vi "transmit-8.6.vi"(0 "can卡类型":u8, 1 "设备索引号":u8, 2 "CAN端口":u8, 4 "单帧发送?":bool=TRUE, 5 "错误输入（无错误）":errorcluster, 6 "ID":u32 format="%x", 7 "SendType":u8, 8 "Data":u8[](array[numeric]), 9 "Eflag":u8=1 format="%x") -> (14 "返回值ID":u32 format="%x", 15 "发送返回值":u32, 16 "发送成功":bool, 19 "错误输出":errorcluster)   [LabVIEW 2013]
uses:
  AutoBurn/Settings/ControlCAN.dll
panel:
  in  "3":u8 format="%x"
  in  "2":u8 format="%x"
  in  "1":u8 format="%x"
  in  "长度":u8=8 format="%x"
  in  "RemoteFlag":u8 format="%x"
  in  "flag":u8 format="%x"
  in  "TimeStamp":u32 format="%x"
  out "VCI_CAN_OBJ_T":T1={"ID"=0, "TimeStamp"=0, "TimeFlag"=0, "SendType"=1, "RemoteFlag"=0, "ExternFlag"=0, "DataLen"=8, 0, 0, 0, 0, 0, 0, 0, 0, 0, 0, 0}
  in  "VCI_CAN_OBJ_T_N":T2(array[cluster])=[{"ID"=0, "TimeStamp"=0, "TimeFlag"=0, "SendType"=1, "RemoteFlag"=0, "ExternFlag"=0, "DataLen"=8, 0, 0, 0, 0, 0, 0, 0, 0, 0, 0, 0}, {"ID"=0, "TimeStamp"=0, "TimeFlag"=0, "SendType"=1, "RemoteFlag"=0, "ExternFlag"=0, "DataLen"=8, 0, 0, 0, 0, 0, 0, 0, 0, 0, 0, 0}, {"ID"=0, "TimeStamp"=0, "TimeFlag"=0, "SendType"=1, "RemoteFlag"=0, "ExternFlag"=0, "DataLen"=8, 0, 0, 0, 0, 0, 0, 0, 0, 0, 0, 0}, {"ID"=0, "TimeStamp"=0, "TimeFlag"=0, "SendType"=1, "RemoteFlag"=0, "ExternFlag"=0, "DataLen"=8, 0, 0, 0, 0, 0, 0, 0, 0, 0, 0, 0}, {"ID"=0, "TimeStamp"=0, "TimeFlag"=0, "SendType"=1, "RemoteFlag"=0, "ExternFlag"=0, "DataLen"=8, 0, 0, 0, 0, 0, 0, 0, 0, 0, 0, 0}, {"ID"=0, "TimeStamp"=0, "TimeFlag"=0, "SendType"=1, "RemoteFlag"=0, "ExternFlag"=0, "DataLen"=8, 0, 0, 0, 0, 0, 0, 0, 0, 0, 0, 0}, {"ID"=0, "TimeStamp"=0, "TimeFlag"=0, "SendType"=1, "RemoteFlag"=0, "ExternFlag"=0, "DataLen"=8, 0, 0, 0, 0, 0, 0, 0, 0, 0, 0, 0}, {"ID"=0, "TimeStamp"=0, "TimeFlag"=0, "SendType"=1, "RemoteFlag"=0, "ExternFlag"=0, "DataLen"=8, 0, 0, 0, 0, 0, 0, 0, 0, 0, 0, 0}, {"ID"=0, "TimeStamp"=0, "TimeFlag"=0, "SendType"=1, "RemoteFlag"=0, "ExternFlag"=0, "DataLen"=8, 0, 0, 0, 0, 0, 0, 0, 0, 0, 0, 0}, {"ID"=0, "TimeStamp"=0, "TimeFlag"=0, "SendType"=1, "RemoteFlag"=0, "ExternFlag"=0, "DataLen"=8, 0, 0, 0, 0, 0, 0, 0, 0, 0, 0, 0}]
  # "说明: TimeStamp 接收到信息帧时的时间标识,从CAN控制器初始化开始计时\n      TimeFlag  是否使用时间标识,为1时TimeStamp有效\n      SendType  发送帧类型 =0时为正常发送\n                           =1时为单次发送\n                           =2时为自发自收\n                           =3时为单次自发自收\n      RemoteFlag 是否为远程帧\n      ExternFlag(Eflag) 是否是扩展帧"
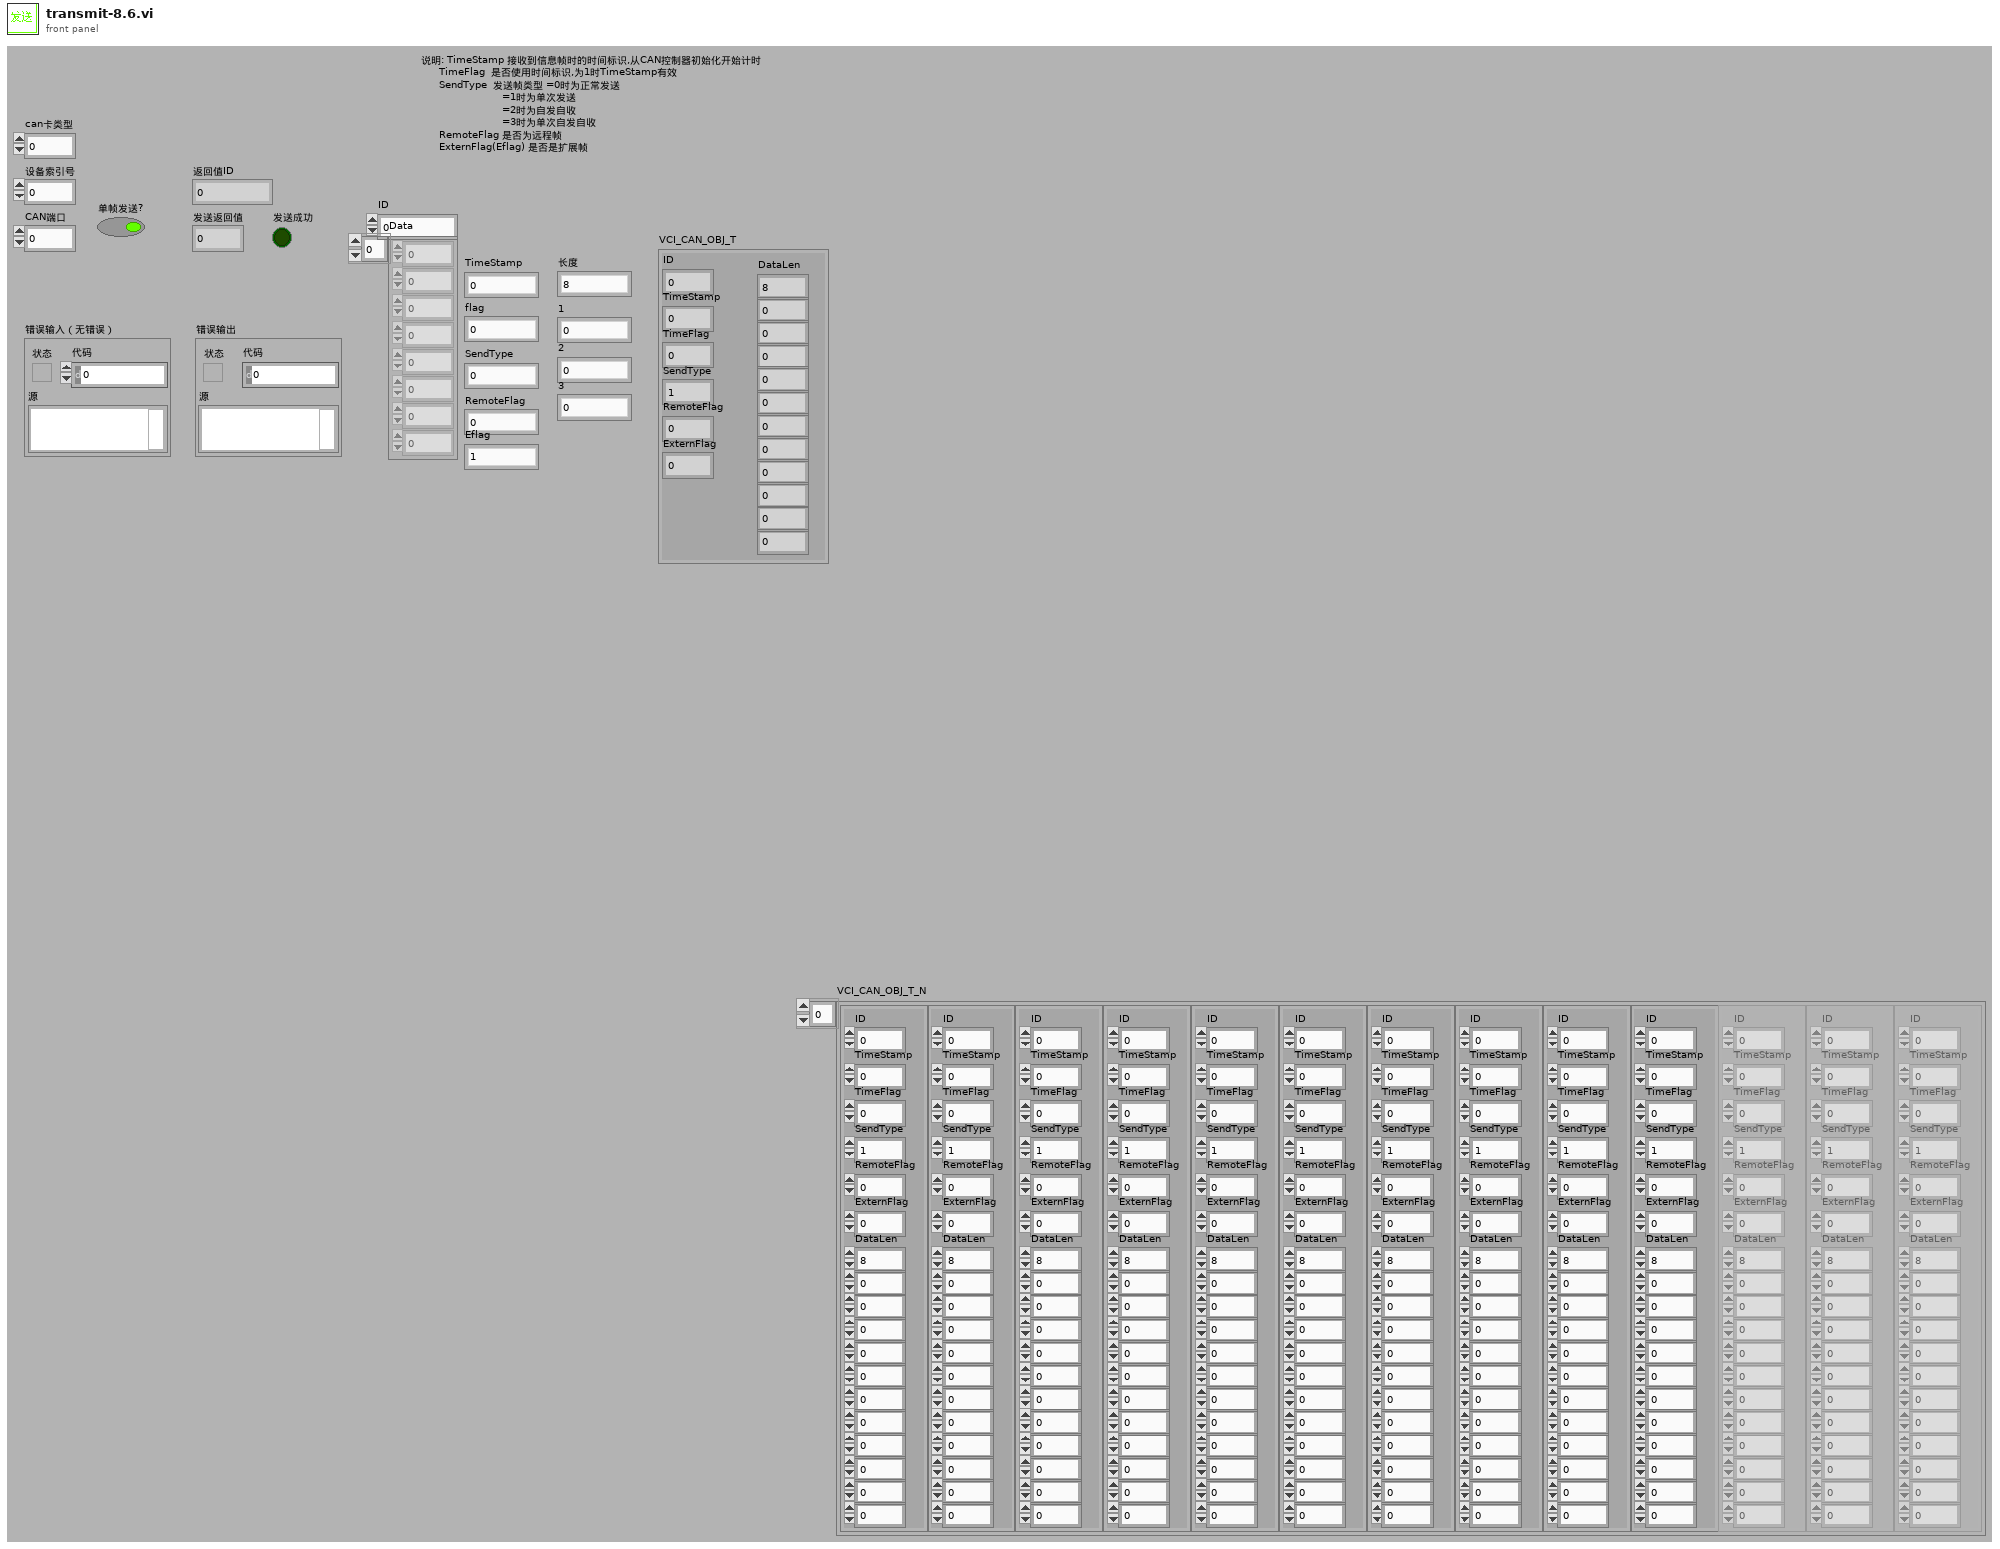
[diagram p1: front panel]
types:
  T1 = cluster{"ID":u32, "TimeStamp":u32, "TimeFlag":u8, "SendType":u8, "RemoteFlag":u8, "ExternFlag":u8, "DataLen":u8, u8, u8, u8, u8, u8, u8, u8, u8, u8, u8, u8}
  T2 = cluster{"ID":u32, "TimeStamp":u32, "TimeFlag":u8, "SendType":u8, "RemoteFlag":u8, "ExternFlag":u8, "DataLen":u8, u8, u8, u8, u8, u8, u8, u8, u8, u8, u8, u8}[]
  T3 = cluster{"ID":u32, "TimeStamp":u32, "flag":u8, "SendType":u8, "RemoteFlag":u8, "Eflag":u8, "长度":u8, "数值":u8, "数值":u8, "数值":u8, "数值":u8, "数值":u8, "数值":u8, "数值":u8, "数值":u8, "1":u8, "2":u8, "3":u8}
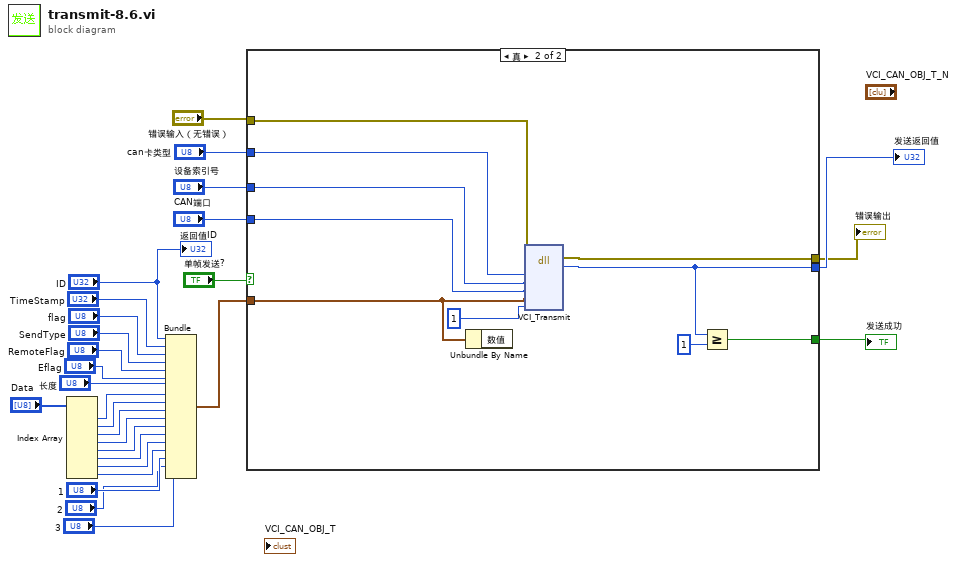
[diagram p0: block diagram]
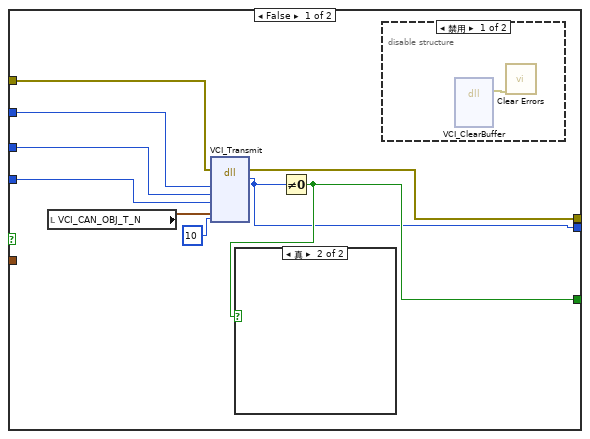
[diagram p2: hidden frame]
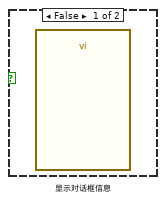
[diagram p4: hidden frame]
diagram:
  n1 = Index Array(array="Data") -> (element #1=w19:u8, element #2=w18:u8, element #3=w17:u8, element #4=w16:u8, element #5=w15:u8, element #6=w14:u8, element #7=w13:u8, element #8=w12:u8)  [unwired: 8 in]
  n2 = Bundle("ID"="ID", "TimeStamp"="TimeStamp", "flag"="flag", "SendType"="SendType", "RemoteFlag"="RemoteFlag", "Eflag"="Eflag", "长度"="长度", "数值"=w19, "数值"=w18, "数值"=w17, "数值"=w16, "数值"=w15, "数值"=w14, "数值"=w13, "数值"=w12, "1"="1", "2"="2", "3"="3") -> (w8:T3)  [unwired: 1 out]
  n3 = case shown="真" "单帧发送?" {
    tunnel: "设备索引号" -> [w34 w42]
    tunnel: "CAN端口" -> [w33 w41]
    tunnel: "can卡类型" -> [w35 w44]
    tunnel: [w29 w43] -> w25
    tunnel: "错误输入（无错误）" -> [w32 w45]
    tunnel: [w31 w46] -> w23
    tunnel: [w30 w47] -> w21
    tunnel: w8 -> [_ w39]
    frame False {
      n4 = local read "VCI_CAN_OBJ_T_N"() -> (w37:T2)
      n5 = dll-call lib="F:/Bluewave New Energy/SVN_Work/AutoTest_TestStand/trunk/AutoTest_TestStand/Driver/ZlgCan/BHN01/AutoBurn/Settings/ControlCAN.dll" fn="VCI_Transmit"(error in=w32, "DeviceType"=w35, "DeviceInd"=w34, "CANInd"=w33, "pSend"=w37, "Len"=u32 10) -> (error out=w31:errorcluster, "返回类型"=w29:u32)  [unwired: 4 in, 4 out]
      n6 = Not Equal To 0?(x=w29) -> (x != 0?=w30:bool)
      n7 = case shown="真" w30 {
        frame False {
          n8 = call "显示对话框信息"() -> ()  [unwired: 3 in, 9 out]
        }
        frame True {
        }
      }
      n9 = disable-structure shown="禁用" {
        frame Disabled {
          n10 = dll-call lib="PTH1abs FBluewave New EnergySVN_WorkAutoTest_TestStandtrunkAutoTest_TestStandDriverZlgCanBHN01è¯»ååæ°data\nkerneldlls\nusbcan.dll" fn="VCI_ClearBuffer"() -> (error out=w38:errorcluster)  [unwired: 5 in, 6 out]
          n11 = call <vilib>:"Clear Errors.vi"("error in (no error)"=w38) -> ()  [unwired: 6 in, 1 out]
        }
        frame Enabled {
        }
      }
    }
    frame True {
      n12 = Unbundle By Name(w39) -> ()  [unwired: 1 out]
      n13 = dll-call lib="F:/Bluewave New Energy/SVN_Work/AutoTest_TestStand/trunk/AutoTest_TestStand/Driver/ZlgCan/BHN01/AutoBurn/Settings/ControlCAN.dll" fn="VCI_Transmit"(error in=w45, "DeviceType"=w44, "DeviceInd"=w42, "CANInd"=w41, "pSend"=w39, "Len"=u32 1) -> (error out=w46:errorcluster, "返回类型"=w43:u32)  [unwired: 4 in, 4 out]
      n14 = Greater Or Equal?(x=w43, y=u32 1) -> (x >= y?=w47:bool)
    }
  }
  "发送成功" <- w21
  "发送返回值" <- w25
  "错误输出" <- w23
  "返回值ID" <- "ID"
